vi "bb.vi"(10 "Matches (Color Pattern Matching 2)":T1(array[cluster]) {"Bounding Box"."y" format="%.2f"; "Bounding Box"."x" format="%.2f"; "Position"."y" format="%.2f"; "Position"."x" format="%.2f"; "Score" format="%.2f"; "Scale" format="%.2f"; "Angle" format="%.2f"}) -> (2 "Array":T2(array[cluster]))   [LabVIEW 2013]
uses:
  <vilib>/imath/engines/lvmath2/RunTimeEngine/ErrorHandling/NIMS_Finalize Error.vi
  <vilib>/imath/engines/lvmath2/RunTimeEngine/NodeEndStatement/NIMS_NodeEndStatement_Output.vi
  <instcachedir>/0/NIMS_NodeEndStatement_Output_53EC0D466D134D7ABD903AC30B43404B.lvgen/NIMS_NodeEndStatement_Output_53EC0D466D134D7ABD903AC30B43404B_010.vi
  <vilib>/imath/engines/lvmath2/RunTimeEngine/RunTimeType/NIMS_RunTimeType_From StrictType (excl LVString).vi
  <instcachedir>/0/NIMS_RunTimeType_From StrictType (excl LVString)_4DEE718D6EB74582AA20236969C084FC.lvgen/NIMS_RunTimeType_From StrictType (excl LVString)_4DEE718D6EB74582AA20236969C084FC_011.vi
  <vilib>/imath/engines/lvmath2/RunTimeEngine/Struct/NIMS_StructSetField.vi
  <vilib>/imath/engines/lvmath2/RunTimeEngine/Struct/NIMS_StructGetField.vi
  <vilib>/imath/engines/lvmath2/RunTimeEngine/RunTimeType/NIMS_RunTimeType_To Numeric.vi
  <instcachedir>/0/NIMS_RunTimeType_To Numeric_4795FB10E831402FABFA341B47E20681.lvgen/NIMS_RunTimeType_To Numeric_4795FB10E831402FABFA341B47E20681_008.vi
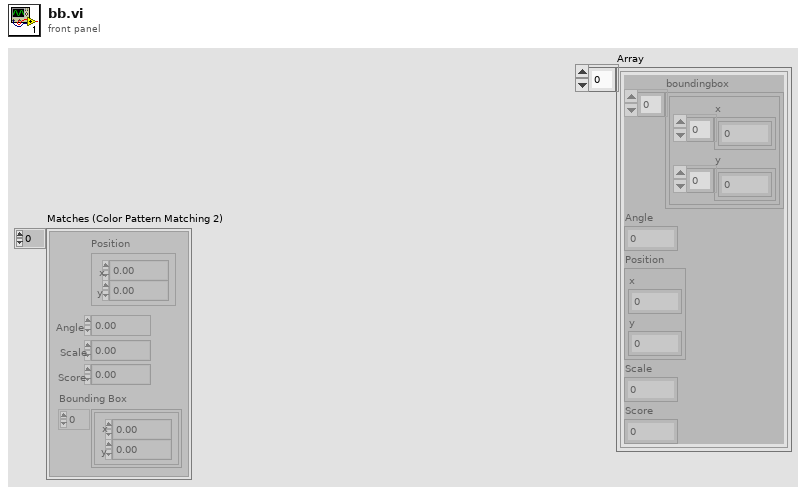
[diagram p1: front panel]
types:
  T1 = cluster{"Position":cluster{"x":sgl, "y":sgl}, "Angle":sgl, "Scale":sgl, "Score":sgl, "Bounding Box":cluster{"x":sgl, "y":sgl}[]}[]
  T2 = cluster{"boundingbox":cluster{"x":sgl[], "y":sgl[]}[], "Angle":sgl, "Position":cluster{"x":sgl, "y":sgl}, "Scale":sgl, "Score":sgl}[]
  T3 = cluster{"boundingbox":cluster{"x":sgl[], "y":sgl[]}[], "Angle":sgl, "Position":cluster{"x":sgl, "y":sgl}, "Scale":sgl, "Score":sgl}
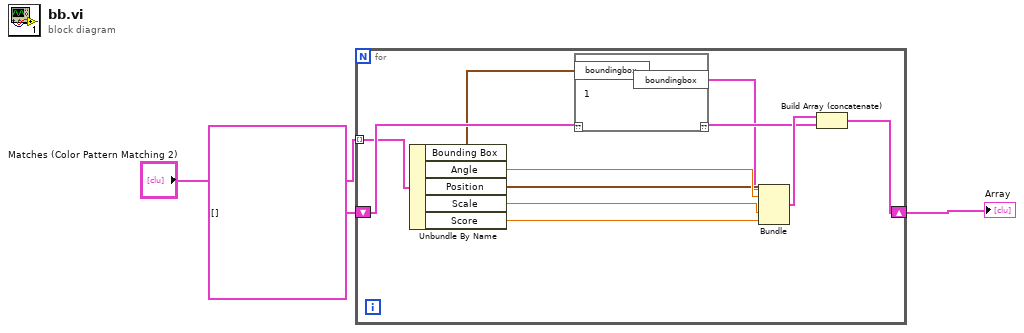
[diagram p0: block diagram]
diagram:
  n1 = for {
    shift-right: [w8] -> w3
    shift-left: T2 [] -> [w7]
    tunnel: "Matches (Color Pattern Matching 2)" -> [w6] mode=indexing
    n2 = Unbundle By Name(w6) -> ("Bounding Box"=w4:cluster{"x":sgl, "y":sgl}[], "Angle"=w13:sgl, "Position"=w12:cluster{"x":sgl, "y":sgl}, "Scale"=w11:sgl, "Score"=w10:sgl)
    n3 = mathscript code="1"("boundingbox"=w4) -> ("boundingbox"=w5:cluster{"x":sgl[], "y":sgl[]}[])  [unwired: 1 in, 1 out]
    n4 = Bundle("boundingbox"=w5, "Angle"=w13, "Position"=w12, "Scale"=w11, "Score"=w10) -> (w9:T3)  [unwired: 1 in]
    n5 = Build Array (concatenate)(w9, w7) -> (w8:T2)
  }
  "Array" <- w3
